vi "Event Structure.vi"() -> ()   [LabVIEW 2011]
panel:
  out "Numeric Control":i32
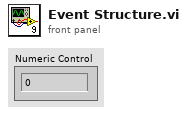
[diagram p1: front panel]
types:
  T1 = cluster{"Operation":enum16{"Cover All"}, "Operation Index (row, column)":cluster{"x":i16, "y":i16}}
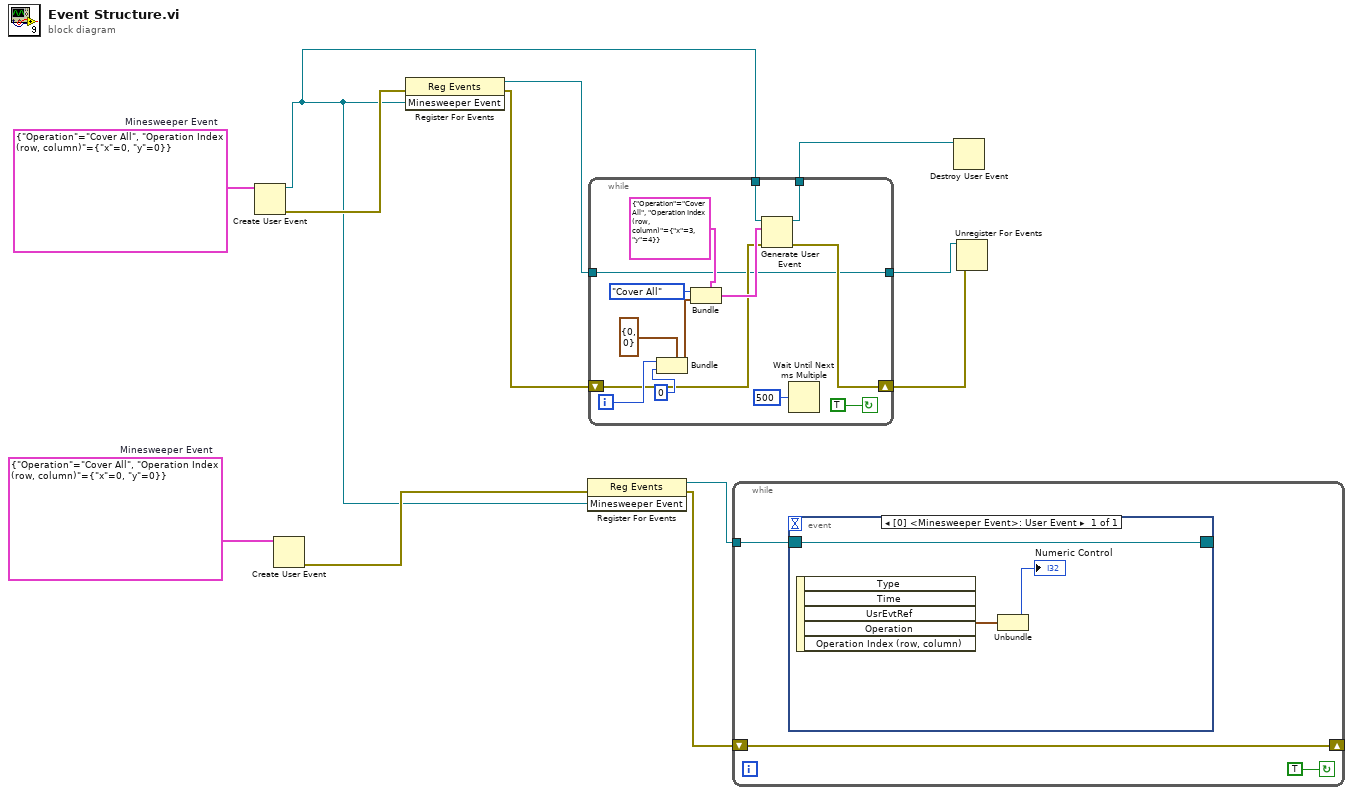
[diagram p0: block diagram]
diagram:
  w3 = T1 {"Operation"=enum."Cover All", "Operation Index (row, column)"={"x"=0, "y"=0}}  # Minesweeper Event
  w12 = T1 {"Operation"=enum."Cover All", "Operation Index (row, column)"={"x"=0, "y"=0}}  # Minesweeper Event
  n1 = Create User Event(user event datatype=w12) -> (user event=w1:refnum<user-event>, error out=w11:errorcluster)  [unwired: 1 in]
  n2 = Create User Event(user event datatype=w3) -> (error out=w2:errorcluster)  [unwired: 1 in, 1 out]
  n3 = register-events(error in=w11, w1) -> (reference out=w8:refnum<event-registration>, error out=w9:errorcluster)  [unwired: 1 in]
  n4 = register-events(error in=w2, w1) -> (reference out=w4:refnum<event-registration>, error out=w5:errorcluster)  [unwired: 1 in]
  n5 = while {
    tunnel: w1 -> [w26]
    tunnel: [w25] -> w10
    shift-right: [w15] -> w6
    shift-left: w9 -> [w16]
    tunnel: w8 -> [w14]
    tunnel: [w14] -> w7
    i -> [w20]
    stop <- TRUE continue-if-true
    n6 = Bundle(cluster=cluster{"x":i16, "y":i16} {"x"=0, "y"=0} ("Operation Index (row, column)"), "x"=w20, "y"=0) -> (w18:cluster{"x":i16, "y":i16})
    n7 = Bundle(cluster=T1 {"Operation"=enum."Cover All", "Operation Index (row, column)"={"x"=3, "y"=4}} ("event data"), "Operation"=enum16{"Cover All"}."Cover All", "Operation Index (row, column)"=w18) -> (w17:T1)
    n8 = Generate User Event(user event=w26, event data cluster=w17, error in=w16) -> (user event out=w25:refnum<user-event>, error out=w15:errorcluster)
    n9 = Wait Until Next ms Multiple(millisecond multiple=u32 500) -> ()  [unwired: 1 out]
  }
  n10 = while {
    shift-right: [w29] -> _
    shift-left: w5 -> [w29]
    tunnel: w4 -> [w28]
    stop <- TRUE continue-if-true
    n11 = event shown="[0] <Minesweeper Event>: User Event" {
      selector: w28 -> [w30]
      dyn-events: [w30] -> _
      timeout: _ -> [_]
      event User Event {
        n12 = event-data() -> ("Operation Index (row, column)"=w32:cluster{"x":i16, "y":i16})  [unwired: 1 in, 4 out]
        n13 = Unbundle(w32) -> ("x"=→"Numeric Control":i16)  [unwired: 1 out]
      }
    }
  }
  n14 = Destroy User Event(user event=w10) -> ()  [unwired: 1 in, 1 out]
  n15 = Unregister For Events(event registration refnum=w7, error in=w6) -> ()  [unwired: 1 out]
